vi "MASTER.vi"() -> ()   [LabVIEW 2013]
doc: "This example demonstrates temperature control and monitoring.\n\nNote:\nBefore start this VI is it necessary:\n\n- preconfigure some specific parameters that are not supported by this driver (e.g. PV-I/O Type, Linearization type, Alarm Input Values... ) by Quick Codes, or by Eurotherm iTools or by instrument front panel controls\n- enter correct VISA Resource Descriptor, Device Address and Baud Rate into front-panel controls"
uses:
  <vilib>/DAQmx/read.llb/DAQmx Read (Analog DBL 1Chan 1Samp).vi
  <vilib>/Utility/file.llb/Write To Spreadsheet File (string).vi
  <vilib>/DAQmx/miscellaneous.llb/DAQmx Fill In Error Info.vi
panel:
  in  "stop":bool
  in  "Tab Control":enum32{"Setup", "QCM", "SetNag O2 Gauge"}(tab)
  in  "Add comments to the data file here and click anywhere outside the comment box to save. \nThe time at which comment is saved is recorded in the data file.":string
  out "Resistance (Ohm)":dbl format="%.6e"
  out "Frequency (Hz)":dbl format="%.6e"
  out "Freq and Resistance Graph 2":T1(graph)
  out "Waveform Chart 2":dbl(graph)
  out "Waveform Chart":cluster{dbl}(graph)
  in  "Baud Rate":i32(ring)=2 items=["2400", "4800", "9600", "19200", "38400", "57600", "115200"]
  in  "Com Port":i32(ring) items=["Com 1", "Com 2", "Com 3", "Com 4", "Com 5", "Com 6", "COM 7", "COM 8", "COM 9", "COM 10", "COM 11", "COM 12", "com 13", "COM 14"]
  out "Torr":dbl
  out "%":dbl
  out "O2 pump voltage (V)":dbl format="%0.2f"
  out "atm":dbl
  # "Configuring Instrument\n \nPlease Wait......\n\nChart will update in 20 sec"
  # "Instructions:\n\nMake sure all instruments are plugged into the correct ports and all instruments are turned on.\n\nRun the Pirani Control software, and make sure the program is configured to save the temp / pressure / gas flow data. \n\nClick the RUN arrow on the toolbar, and wait for instruments to begin recording.\n\nTo end, click \"END PROGRAM AND SAVE DATA\". DO NOT press the STOP button on the toolbar."
  # "COMMENT BOX"
  # "BEFORE YOU RUN THIS VI:\n1. Turn on SetNag and get to 800C\n2. Turn on QCM and plug into corrent COM.\n3. Plug in USB DAQ 6008 and comment to SetNag"
  # "O2 Partial Pressure"
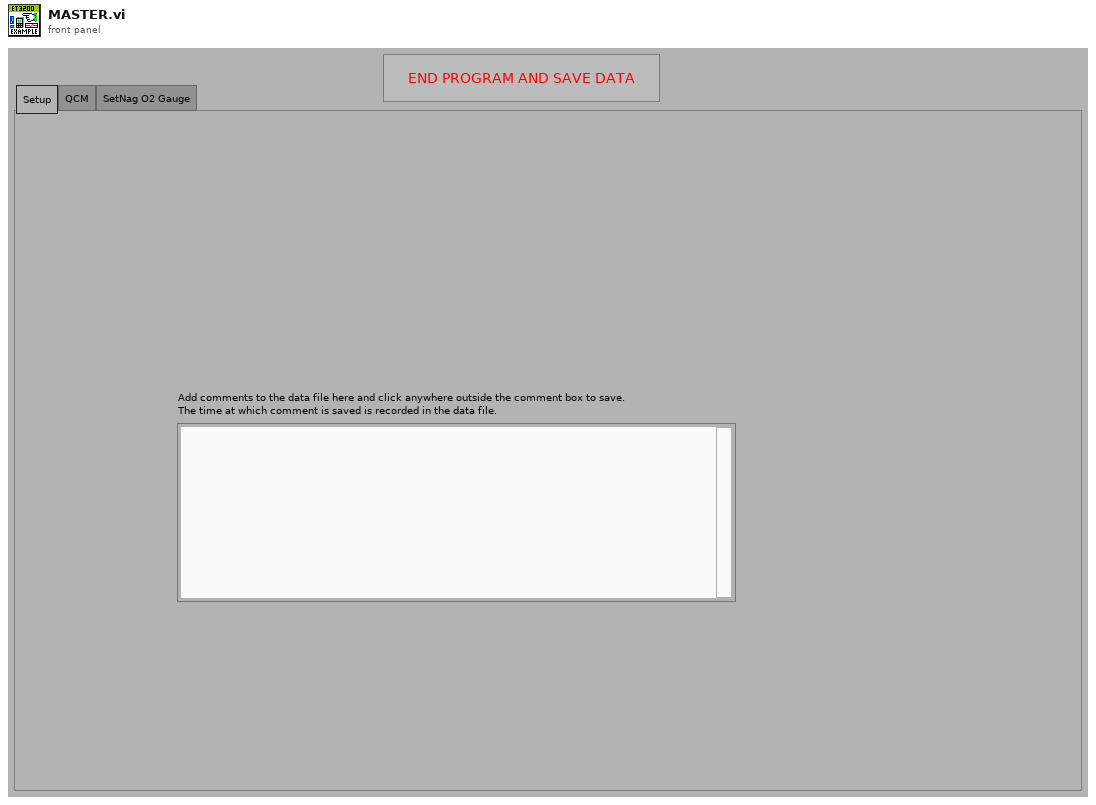
[diagram p1: front panel]
types:
  T1 = cluster{"XY chart data":cluster{"x":dbl, "y":dbl}[]}[]
  T2 = enum16{"no parity", "odd parity", "even parity", "mark parity", "space parity"}
  T3 = cluster{"timestamp out":dbl, "Frequency out":dbl}
  T4 = cluster{"timestamp out":dbl, "Resistance out":dbl}
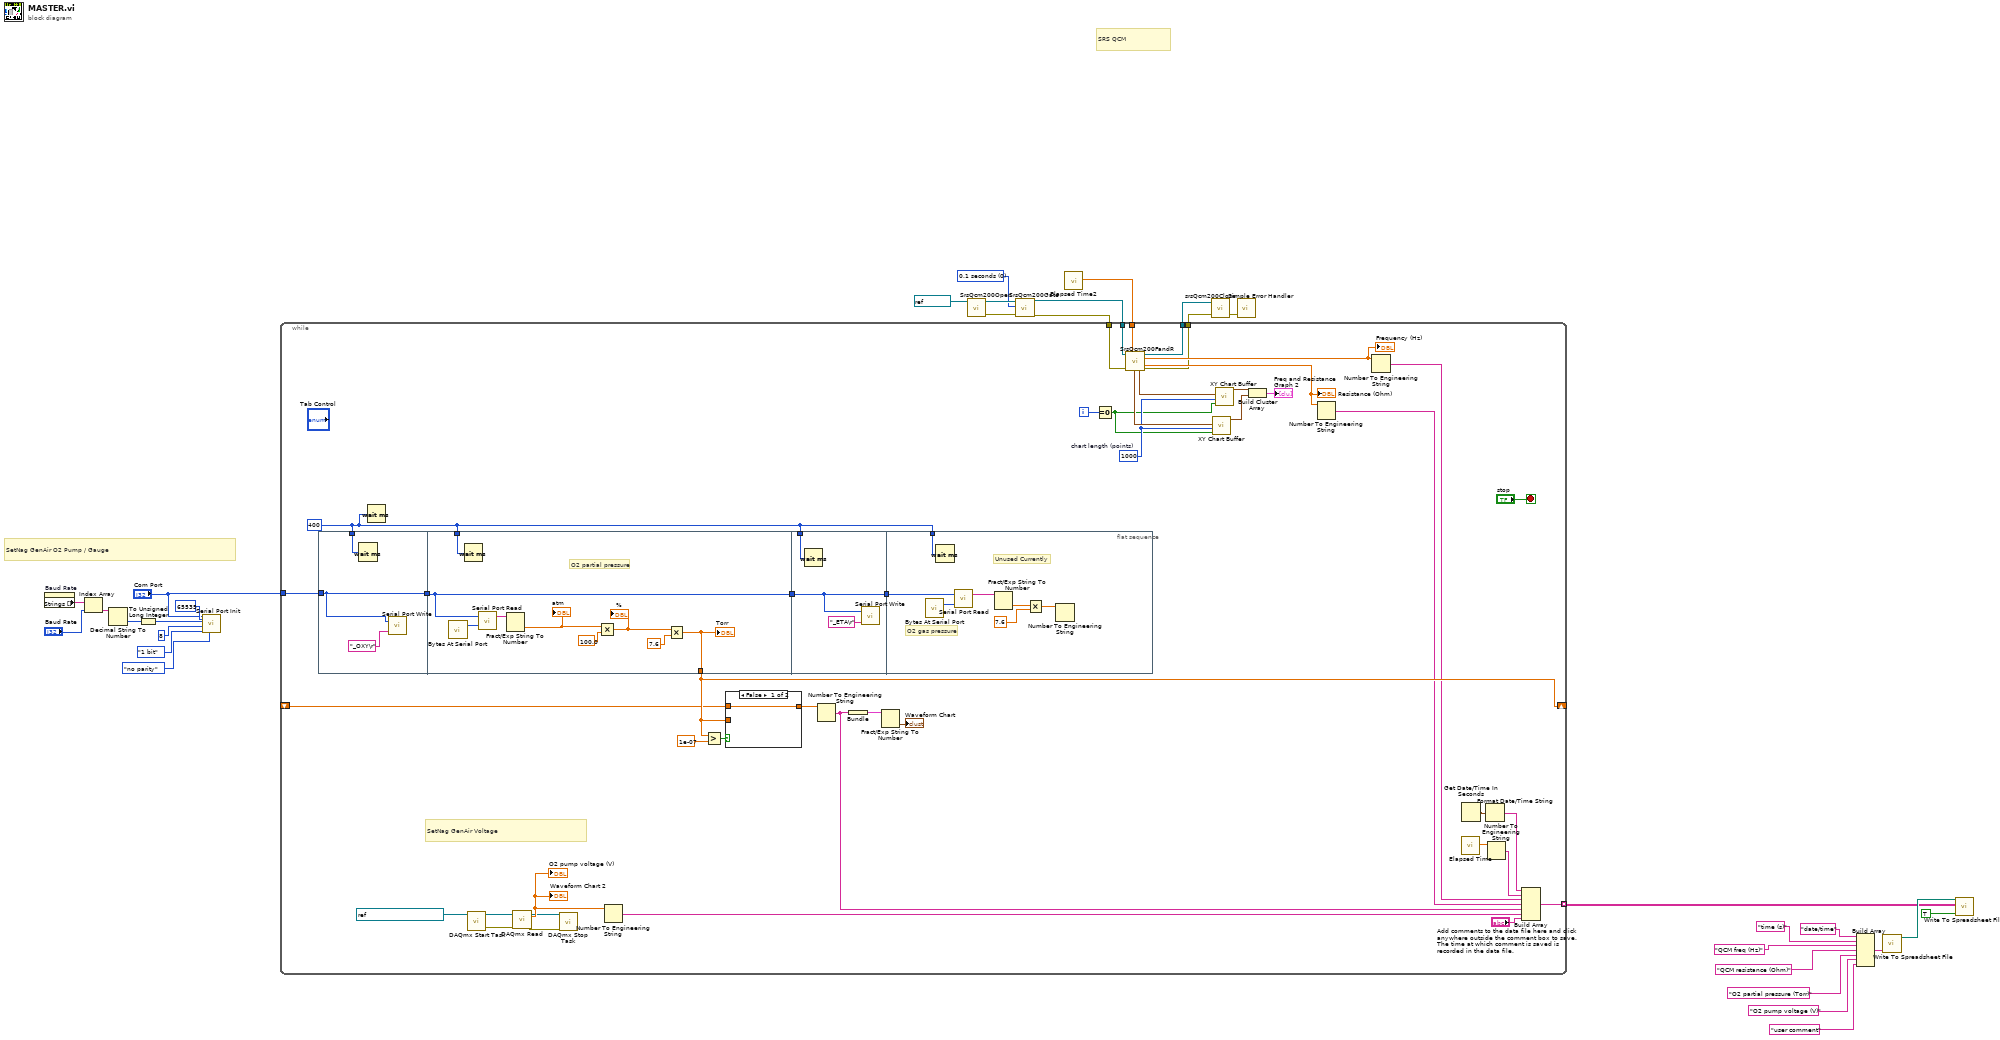
[diagram p0: block diagram]
diagram:
  w8 = u16 0 items=["0.1 seconds", "1.0 seconds", "10.0 seconds"] ("Gate in")
  # "SRS QCM"
  # "SetNag GenAir O2 Pump / Gauge"
  n1 = property on="Baud Rate" class="Ring (strict)"() -> ("Strings []"=w20:string[])  [unwired: 2 in, 2 out]
  n2 = Index Array(array=w20, index="Baud Rate") -> (element=w21:string)
  n3 = Decimal String To Number(string=w21) -> (number=w19:i32)  [unwired: 2 in, 1 out]
  n4 = To Unsigned Long Integer(number=w19) -> (unsigned 32bit integer=w22:u32)
  n5 = call <vilib>:"Serial Port Init.vi"("parity"=T2."no parity", "buffer size"=u16 65535, "stop bits"=enum16{"1 bit", "1.5 bits", "2 bits"}."1 bit", "data bits"=u16 8, "baud rate"=w22, "port number"="Com Port") -> ()  [unwired: 1 in, 1 out]
  n6 = call <instrlib>:"SrsQcm200Open.vi"("VISA in"=refnum<visa-resource-name> "COM6") -> ("error out"=w12:errorcluster, "VISA out"=w11:refnum<visa-resource-name>)  [unwired: 4 in]
  n7 = call <instrlib>:"SrsQcm200Gate.vi"("VISA in"=w11, "Gate in"=w8, "error in (no error)"=w12) -> ("VISA out"=w4:refnum<visa-resource-name>, "error out"=w3:errorcluster)  [unwired: 14 in, 1 out]
  n8 = call "Elapsed Time2"() -> ("Elapsed Time (s)"=w5:dbl)  [unwired: 12 in, 7 out]
  n9 = while {
    tunnel: [w74] -> w28 mode=indexing
    tunnel: "Com Port" -> [w68]
    shift-right: [w50] -> _
    shift-left: _ -> [w49]
    tunnel: [w38] -> w7
    tunnel: [w37] -> w6
    tunnel: w5 -> [w36]
    tunnel: w4 -> [w35]
    tunnel: w3 -> [w34]
    i -> [w39]
    stop <- "stop" stop-if-true
    w46 = 1000  # chart length (points)
    w63 = u32 400 ("milliseconds to wait")
    # "SetNag GenAir Voltage"
    n10 = flat-sequence {
      tunnel: [w78] -> w71
      tunnel: w63 -> [w80]
      tunnel: w68 -> [w78]
      tunnel: w71 -> [w86]
      tunnel: w63 -> [w88]
      tunnel: [w86] -> w65
      tunnel: [w83] -> w50
      tunnel: w65 -> [w91]
      tunnel: [w91] -> w64
      tunnel: w63 -> [w90]
      tunnel: w64 -> [w97]
      tunnel: w63 -> [w96]
      frame #0 {
        n11 = Wait (ms)(milliseconds to wait=w80) -> ()  [unwired: 1 out]
        n12 = call <vilib>:"Serial Port Write.vi"("string to write"="_OXY\r" ("O2 partial press"), "port number"=w78) -> ()  [unwired: 1 out]
      }
      frame #1 {
        # "O2 partial pressure"
        n13 = call <vilib>:"Bytes At Serial Port.vi"() -> ("byte count"=w89:u32)  [unwired: 1 in, 1 out]
        n14 = Wait (ms)(milliseconds to wait=w88) -> ()  [unwired: 1 out]
        n15 = call <vilib>:"Serial Port Read.vi"("requested byte count"=w89, "port number"=w86) -> ("string read"=w87:string)  [unwired: 1 out]
        n16 = Fract/Exp String To Number(string=w87) -> (number=w84:dbl)  [unwired: 3 in, 1 out]
        "atm" <- w84
        n17 = Multiply(x=w84, y=100.0) -> (x*y=w81:dbl)
        "%" <- w81
        n18 = Multiply(x=w81, y=7.6) -> (x*y=w83:dbl)
        "Torr" <- w83
      }
      frame #2 {
        n19 = Wait (ms)(milliseconds to wait=w90) -> ()  [unwired: 1 out]
        n20 = call <vilib>:"Serial Port Write.vi"("string to write"="_ETA\r" ("O2 partial press"), "port number"=w91) -> ()  [unwired: 1 out]
      }
      frame #3 {
        # "Unused Currently"
        # "O2 gas pressure"
        n21 = call <vilib>:"Bytes At Serial Port.vi"() -> ("byte count"=w98:u32)  [unwired: 1 in, 1 out]
        n22 = Wait (ms)(milliseconds to wait=w96) -> ()  [unwired: 1 out]
        n23 = call <vilib>:"Serial Port Read.vi"("requested byte count"=w98, "port number"=w97) -> ("string read"=w99:string)  [unwired: 1 out]
        n24 = Fract/Exp String To Number(string=w99) -> (number=w93:dbl)  [unwired: 3 in, 1 out]
        n25 = Multiply(x=w93, y=7.6) -> (x*y=w94:dbl)
        n26 = Number To Engineering String(4:w94) -> ()  [unwired: 3 in, 1 out]
      }
    }
    n27 = Wait (ms)(milliseconds to wait=w63) -> ()  [unwired: 1 out]
    n28 = call <vilib>:"DAQmx Start Task.vi"("task/channels in"=refnum<k21> "SetNag_Pump_Voltage") -> ("task out"=w61:refnum<k21>, "error out"=w60:errorcluster)  [unwired: 13 in]
    n29 = call-poly <vilib>:"DAQmx Read.vi"("task/channels in"=w61, "error in"=w60) -> ("task out"=w59:refnum<k21>, "data"=w67:dbl, "error out"=w58:errorcluster)  [unwired: 11 in]
    "Waveform Chart 2" <- w67
    "O2 pump voltage (V)" <- w67
    n30 = call <vilib>:"DAQmx Stop Task.vi"("task/channels in"=w59, "error in"=w58) -> ()  [unwired: 12 in, 2 out]
    n31 = Number To Engineering String(4:w67) -> (0:w54:string)  [unwired: 3 in]
    n32 = Greater?(x=w50, y=1e-07) -> (0:w52:bool)
    n33 = case shown="False" w52 {
      tunnel: [w76 w77] -> w51
      tunnel: w50 -> [_ w77]
      tunnel: w49 -> [w76 _]
      frame False {
      }
      frame True {
      }
    }
    n34 = Number To Engineering String(4:w51) -> (0:w57:string)  [unwired: 3 in]
    n35 = Bundle(w57) -> (w66:cluster{string})  [unwired: 1 in]
    n36 = Fract/Exp String To Number(string=w66) -> (number=→"Waveform Chart":cluster{dbl})  [unwired: 3 in, 1 out]
    n37 = Equal To 0?(x=w39) -> (x = 0?=w42:bool)
    n38 = call <instrlib>:"SrsQcm200FandR.vi"("VISA in"=w35, "Reference time in"=w36, "error in (no error)"=w34) -> ("VISA out"=w37:refnum<visa-resource-name>, "Frequency out"=w41:dbl, "Resistance out"=w40:dbl, "F vs T out"=w48:T3, "R vs T out"=w47:T4, "error out"=w38:errorcluster)  [unwired: 6 in, 1 out]
    "Frequency (Hz)" <- w41
    "Resistance (Ohm)" <- w40
    n39 = call <instrlib>:"XY Chart Buffer.vi"("clear first (no:F)"=w42, "chart length (points)"=w46, "new point"=w48) -> ("XY chart data"=w44:cluster{"x":dbl, "y":dbl}[])  [unwired: 8 in]
    n40 = call <instrlib>:"XY Chart Buffer.vi"("clear first (no:F)"=w42, "chart length (points)"=w46, "new point"=w47) -> ("XY chart data"=w45:cluster{"x":dbl, "y":dbl}[])  [unwired: 8 in]
    n41 = Build Cluster Array(w45, w44) -> (→"Freq and Resistance Graph 2":T1)
    n42 = Number To Engineering String(4:w40) -> (0:w32:string)  [unwired: 3 in]
    n43 = Number To Engineering String(4:w41) -> (0:w33:string)  [unwired: 3 in]
    n44 = call "Elapsed Time"() -> ("Elapsed Time (s)"=w73:dbl)  [unwired: 12 in, 7 out]
    n45 = Get Date/Time In Seconds() -> (seconds since 1Jan1904=w75:timestamp)
    n46 = Format Date/Time String(seconds (now)=w75) -> (date/time string=w55:string)  [unwired: 2 in]
    n47 = Number To Engineering String(4:w73) -> (0:w56:string)  [unwired: 3 in]
    n48 = Build Array(w55, w56, w33, w32, w57, w54, "Add comments to the data file here and click anywhere outside the comment box to save. \nThe time at which comment is saved is recorded in the data file.") -> (w74:string[])
  }
  n49 = call <instrlib>:"srsQcm200Close.vi"("error in"=w7, "Visa in"=w6) -> ("error out"=w9:errorcluster)  [unwired: 3 in]
  n50 = call <vilib>:"Simple Error Handler.vi"("error in (no error)"=w9) -> ()  [unwired: 4 in, 5 out]
  n51 = Build Array("date/time", "time (s)", "QCM freq (Hz)", "QCM resistance (Ohm)", "O2 partial pressure (Torr)" ("element"), "O2 pump voltage (V)" ("element"), "user comment" ("element")) -> (w30:string[])
  n52 = call-poly <vilib>:"Write To Spreadsheet File.vi"("1D data"=w30) -> ("new file path (Not A Path if cancelled)"=w29:path)  [unwired: 7 in]
  n53 = call-poly <vilib>:"Write To Spreadsheet File.vi"("append to file? (new file:F)"=TRUE, "2D data"=w28, "file path (dialog if empty)"=w29) -> ()  [unwired: 5 in, 1 out]
